vi "dequeue_command_by_dim_name.vi"(8 "error in (no error)":errorcluster caption="错误输入（无错误）", 10 "name":string, 11 "MotorSystem 输入":refnum<class "MotorSystem.lvclass">) -> (0 "error out":errorcluster caption="错误输出", 2 "command":cluster{"cmd":T1, "cmd data":variant}, 3 "MotorSystem 输出":refnum<class "MotorSystem.lvclass">)   [LabVIEW 2016, in "MotionControl_UFO_3DOF.lvlib" / "MotorSystem.lvclass"]
uses:
  <userlib>/MotionControl_UFO_3DOF/MotorSystem/MotorSystem.lvclass
  <userlib>/MotionControl_UFO_3DOF/OneMotion/cmd_motion.ctl
  <userlib>/MotionControl_UFO_3DOF/MotorSystem/MotorSystem.lvclass/MotorSystem.ctl
  <userlib>/MotionControl_UFO_3DOF/OneMotion/OneMotion.lvclass
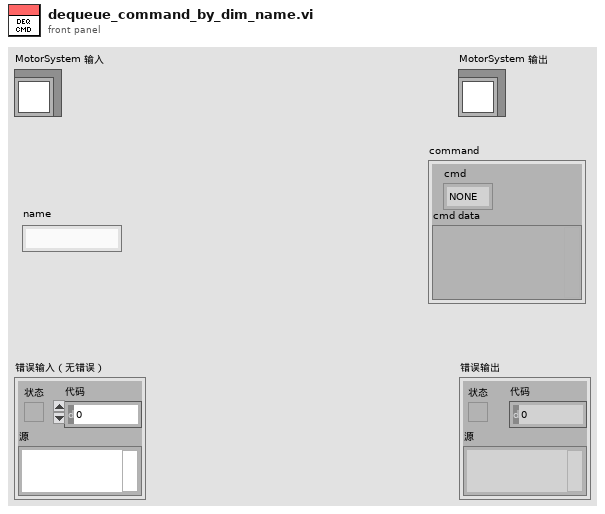
[diagram p1: front panel]
types:
  T1 = typedef "MotionControl_UFO_3DOF.lvlib/OneMotion.lvclass/cmd_motion.ctl" = enum16{"NONE", "MOVE_MOTION", "EXIT", "STP_MOTION", "SPEED_MOTION", "WAIT_FOR_S3", "WAIT_A_TIME", "SKIP", "RETRACT_BEFORE_ROT"}
  T2 = typedef "MotionControl_UFO_3DOF.lvlib/MotorSystem.lvclass/MotionCluster.ctl" = cluster{"OneMotion.lvclass":refnum<class "OneMotion.lvclass">, "connected?":bool, "default enabled?":bool, "enabled?":bool}
  T3 = cluster{"complete dimension names":string[], "dimension names cluster ":cluster{"name 1":string, "name 2":string, "name 3":string}}
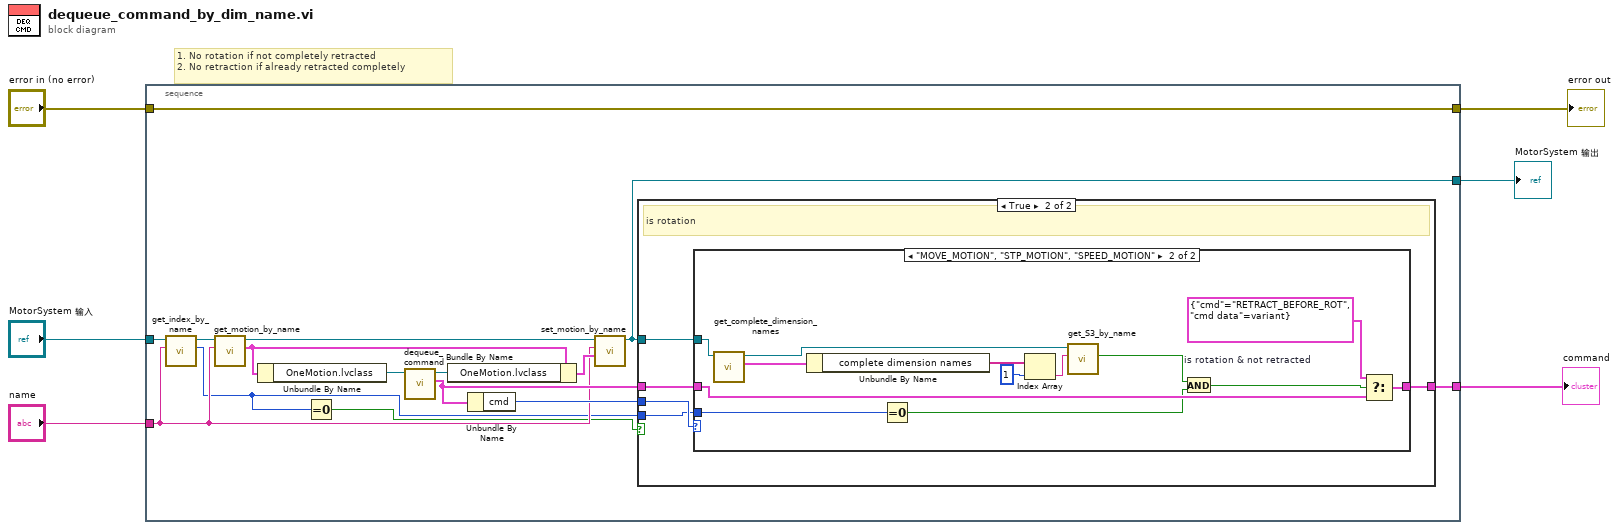
[diagram p0: block diagram]
diagram:
  # "1. No rotation if not completely retracted\n2. No retraction if already retracted completely"
  n1 = stacked-sequence {
    tunnel: [w20] -> w6
    tunnel: [w10] -> w4
    tunnel: "MotorSystem 输入" -> [w21]
    tunnel: "name" -> [w9]
    tunnel: [w13] -> w2
    tunnel: "error in (no error)" -> [w20]
    frame #0 {
      n2 = call <userlib>:"get_index_by_name.vi"("name"=w9, "MotorSystem 输入"=w21) -> ("index (0-based)"=w8:u32, "MotorSystem 输出"=w19:refnum<class "MotorSystem.lvclass">)  [unwired: 7 in, 1 out]
      n3 = call <userlib>:"get_motion_by_name.vi"("name"=w9, "MotorSystem in"=w19) -> ("motion cluster"=w14:T2, "MotorSystem out"=w15:refnum<class "MotorSystem.lvclass">)  [unwired: 7 in, 1 out]
      n4 = Unbundle By Name(w14) -> ("OneMotion.lvclass"=w18:refnum<class "OneMotion.lvclass">)
      n5 = Equal To 0?(x=w8) -> (x = 0?=w7:bool)
      n6 = call <userlib>:"dequeue_command.vi"("OneMotion输入"=w18) -> ("command"=w12:cluster{"cmd":T1, "cmd data":variant}, "OneMotion输出"=w17:refnum<class "OneMotion.lvclass">)  [unwired: 8 in, 1 out]
      n7 = Bundle By Name(cluster=w14, "OneMotion.lvclass"=w17) -> (w16:T2)
      n8 = Unbundle By Name(w12) -> ("cmd"=w11:T1)
      n9 = call <userlib>:"set_motion_by_name.vi"("簇"=w16, "name"=w9, "MotorSystem输入"=w15) -> ("MotorSystem输出"=w10:refnum<class "MotorSystem.lvclass">)  [unwired: 7 in, 1 out]
      n10 = case shown="True" w7 {
        tunnel: [w22 w27] -> w13
        tunnel: w12 -> [w22 w26]
        tunnel: w11 -> [_ w25]
        tunnel: w10 -> [_ w24]
        tunnel: w8 -> [_ w23]
        frame False {
        }
        frame True {
          # "is rotation"
          n11 = case shown="\"MOVE_MOTION\", \"STP_MOTION\", \"SPEED_MOTION\"" w25 {
            tunnel: [w28 w40] -> w27
            tunnel: w26 -> [w28 w39]
            tunnel: w23 -> [_ w36]
            tunnel: w24 -> [_ w35]
            frame Default {
            }
            frame "MOVE_MOTION", "STP_MOTION", "SPEED_MOTION" {
              n12 = call <userlib>:"get_complete_dimension_names.vi"("MotorSystem输入"=w35) -> ("dimension names"=w32:T3, "MotorSystem输出"=w33:refnum<class "MotorSystem.lvclass">)  [unwired: 8 in, 1 out]
              n13 = Unbundle By Name(w32) -> ("complete dimension names"=w31:string[])
              n14 = Equal To 0?(x=w36) -> (x = 0?=w38:bool)
              n15 = Index Array(array=w31, index=1) -> (element=w29:string)
              n16 = call <userlib>:"get_S3_by_name.vi"("name"=w29, "MotorSystem in"=w33) -> ("S3"=w34:bool)  [unwired: 7 in, 2 out]
              n17 = And "is rotation & not retracted"(x=w34, y=w38) -> (x .and. y?=w37:bool)
              n18 = Select(t=cluster{"cmd":T1, "cmd data":variant} {"cmd"=enum."RETRACT_BEFORE_ROT", "cmd data"=variant} ("command"), s=w37, f=w39) -> (s? t:f=w40:cluster{"cmd":T1, "cmd data":variant})
            }
          }
        }
      }
    }
  }
  "error out" <- w6
  "MotorSystem 输出" <- w4
  "command" <- w2
